vi "Stop Core.vi"(10 "final error code":i32, 11 "Assert Display in":refnum<class "Assert Display.lvclass">) -> (3 "Assert Display out":refnum<class "Assert Display.lvclass">)   [LabVIEW 2016, in "Assert API Components.lvlib" / "Assert Display.lvlib" / "Assert Display.lvclass"]
doc: "(<B>Filename</B>: Actor Framework.lvlib:Actor.lvclass:Stop Core.vi)\n\nDefines what the actor does before it stops. Use the <B>final error code</B> input to determine whether the actor shut down in response to an error.\n\nBy default, this method does nothing. A descendant class may override it to define behavior, such as shutting down any processes the actor initiated in its override of the Actor Core method."
uses:
  Assert Display.lvclass
  Assert Display.lvclass/Assert Display.ctl
  <vilib>/ActorFramework/Stop Msg/Stop Msg.lvclass/Stop Msg.ctl
  <vilib>/ActorFramework/Message Enqueuer/Message Enqueuer.lvclass/Message Enqueuer.ctl
  <vilib>/ActorFramework/Stop Msg/Send Emergency Stop.vi
  <vilib>/ActorFramework/Stop Msg/Send Normal Stop.vi
  <vilib>/ActorFramework/Message Enqueuer/Enqueue Critical.vi
  <vilib>/ActorFramework/Message Enqueuer/Enqueue.vi
  <vilib>/ActorFramework/Stop Msg/Stop Msg.lvclass
  C:/Program Files (x86)/National Instruments/LabVIEW 2016/vi.lib/ActorFramework/Message/Message.lvclass
  <vilib>/Utility/LVClass/Get LV Class Name.vi
  <resource>/AFDebug/Generate Trace for Message.vi
  <vilib>/ActorFramework/Message Priority Queue/Priority Enqueue.vi
  Base UI Actor/Base UI Actor/Base UI Actor.lvclass
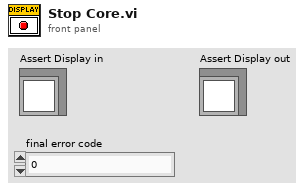
[diagram p1: front panel]
types:
  T1 = typedef "Assert API Components.lvlib/Display Type.ctl" = enum16{"Local", "Network"}
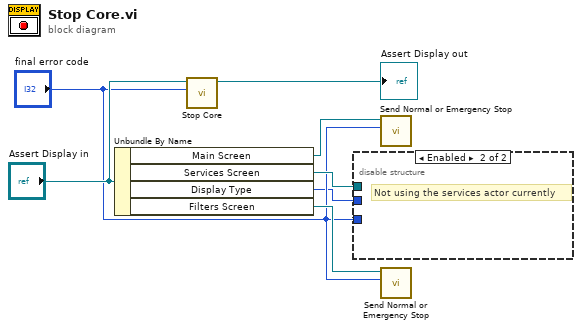
[diagram p0: block diagram]
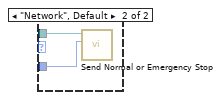
[diagram p3: hidden frame]
diagram:
  n1 = Unbundle By Name("Assert Display in") -> ("Main Screen"=w5:refnum<class "Message Enqueuer.lvclass">, "Services Screen"=w4:refnum<class "Message Enqueuer.lvclass">, "Display Type"=w1:T1, "Filters Screen"=w3:refnum<class "Message Enqueuer.lvclass">)
  n2 = call-parent "Stop Core.vi"("final error code"="final error code", "Base UI Actor in"="Assert Display in") -> ("Base UI Actor out"=→"Assert Display out":refnum<class "Assert Display.lvclass">)  [unwired: 9 in]
  n3 = disable-structure shown="Enabled" {
    disable-tunnel: w4 -> [w10 _]
    disable-tunnel: "final error code" -> [w9 _]
    disable-tunnel: w1 -> [w8 _]
    frame Disabled {
      n4 = case shown="\"Local\"" w8 {
        tunnel: w10 -> [_ w12]
        tunnel: w9 -> [_ w11]
        frame "Local" {
        }
        frame "Network", Default {
          n5 = call <vilib>:"Send Normal or Emergency Stop.vi"("final error code"=w11, "Message Enqueuer"=w12) -> ()  [unwired: 9 in, 1 out]
        }
      }
    }
    frame Enabled {
      # "Not using the services actor currently"
    }
  }
  n6 = call <vilib>:"Send Normal or Emergency Stop.vi"("final error code"="final error code", "Message Enqueuer"=w5) -> ()  [unwired: 9 in, 1 out]
  n7 = call <vilib>:"Send Normal or Emergency Stop.vi"("final error code"="final error code", "Message Enqueuer"=w3) -> ()  [unwired: 9 in, 1 out]
